vi "_017.vi"() -> ()   [LabVIEW 2024]
panel:
  out "output cluster":T1
  in  "String":string
  in  "Boolean":bool
  in  "Numeric":dbl
  out "String":string
  out "Boolean":bool
  out "Numeric":dbl
  in  "Cluster":T2
  out "output cluster":T2
  in  "String":string
  in  "Boolean":bool
  in  "Numeric":dbl
  out "String":string
  out "Boolean":bool
  out "Numeric":dbl
  in  "Cluster":T2
  # "Cluster ( Functions ) :"
  # "Unbundle By Name :"
  # "Bundle By Name :"
  # "Unbundle :"
  # "Bundle :"
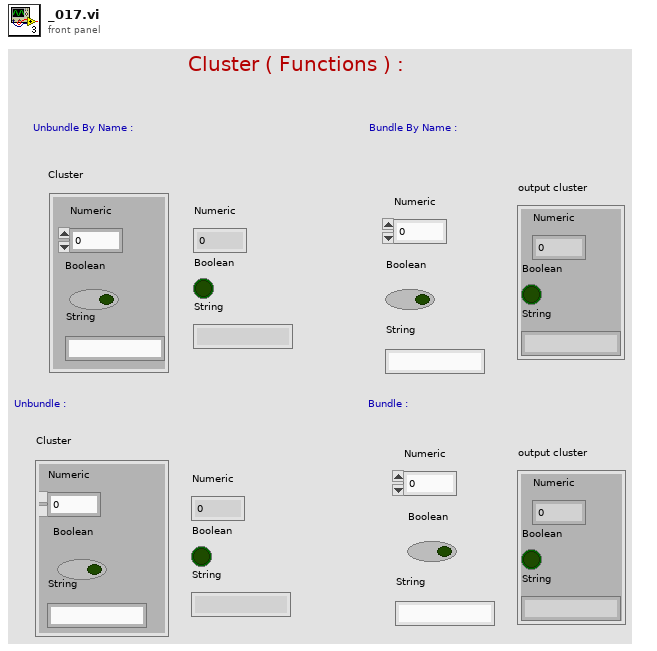
[diagram p1: front panel]
types:
  T1 = cluster{"Numeric ":dbl, "Boolean ":bool, "String":string}
  T2 = cluster{"Numeric":dbl, "Boolean":bool, "String":string}
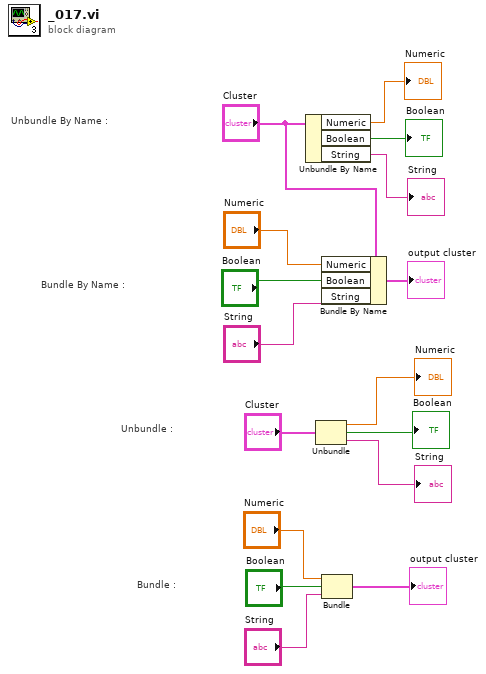
[diagram p0: block diagram]
diagram:
  # "Bundle :"
  # "Unbundle :"
  # "Bundle By Name :"
  # "Unbundle By Name :"
  n1 = Unbundle By Name("Cluster") -> ("Numeric"=→"Numeric":dbl, "Boolean"=→"Boolean":bool, "String"=→"String":string)
  n2 = Unbundle("Cluster") -> ("Numeric"=→"Numeric":dbl, "Boolean"=→"Boolean":bool, "String"=→"String":string)
  n3 = Bundle By Name(cluster="Cluster", "Numeric"="Numeric", "Boolean"="Boolean", "String"="String") -> (→"output cluster":T2)
  n4 = Bundle("Numeric"="Numeric", "Boolean"="Boolean", "String"="String") -> (→"output cluster":T2)  [unwired: 1 in]
